vi "题目4.vi"   [LabVIEW 2017]
uses:
  <vilib>/Utility/file.llb/Write Delimited Spreadsheet (DBL).vi
  <vilib>/measure/NI_MABase.lvlib
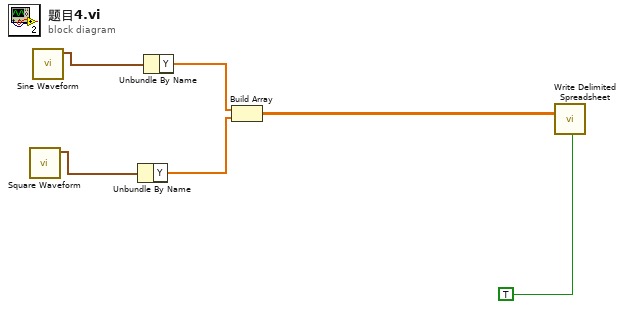
[diagram p0: block diagram]
diagram:
  n1 = call <vilib>:"Square Waveform.vi"() -> ("signal out"=w6:waveform(dbl))  [unwired: 10 in, 1 out]
  n2 = call <vilib>:"Sine Waveform.vi"() -> ("signal out"=w5:waveform(dbl))  [unwired: 10 in, 1 out]
  n3 = Unbundle By Name(w6) -> ("Y"=w3:dbl[])
  n4 = Unbundle By Name(w5) -> ("Y"=w4:dbl[])
  n5 = Build Array(w4, w3) -> (w1:dbl[][])
  n6 = call-poly <vilib>:"Write Delimited Spreadsheet.vi"("2D data"=w1, "append to file? (new file:F)"=TRUE) -> ()  [unwired: 12 in, 2 out]
